vi "Generate Joint Trajectory (Int).vi"(4 "end joint velocities":dbl[](array[numeric]), 6 "start joint velocities":dbl[](array[numeric]), 7 "intermediate points":i32, 8 "error in (no error)":errorcluster, 10 "end joint positions":dbl[](array[numeric]), 11 "start joint positions":dbl[](array[numeric])) -> (0 "error out":errorcluster, 1 "joint acceleration trajectory":dbl[][](array[numeric]), 2 "joint velocity trajectory":dbl[][](array[numeric]), 3 "joint position trajectory":dbl[][](array[numeric]))   [LabVIEW 2017, in "NI_Kinematics.lvlib"]
doc: "Generates joint angles, velocities, and accelerations along a smooth trajectory between two points in joint space. Wire data to the <B>intermediate points</B> input to determine the polymorphic instance to use or manually select the instance.\n\n<B>.m file:</B> jtraj"
uses:
  <vilib>/robotics/Kinematics/NI_Kinematics.lvlib
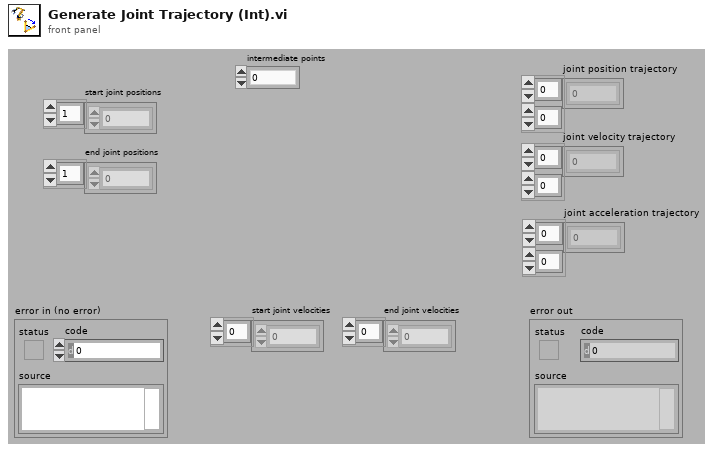
[diagram p1: front panel]
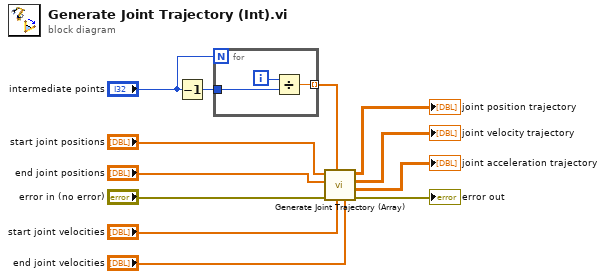
[diagram p0: block diagram]
diagram:
  n1 = Decrement(x="intermediate points") -> (x-1=w7:i32)
  n2 = for {
    N: "intermediate points" -> [_]
    tunnel: w7 -> [w15]
    tunnel: [w13] -> w5 mode=indexing
    i -> [w14]
    n3 = Divide(x=w14, y=w15) -> (x/y=w13:dbl)
  }
  n4 = call <vilib>:"Generate Joint Trajectory (Array).vi"("end joint velocities"="end joint velocities", "start joint velocities"="start joint velocities", "intermediate points"=w5, "error in (no error)"="error in (no error)", "end joint positions"="end joint positions", "start joint positions"="start joint positions") -> ("error out"=→"error out":errorcluster, "joint acceleration trajectory"=→"joint acceleration trajectory":dbl[][], "joint velocity trajectory"=→"joint velocity trajectory":dbl[][], "joint position trajectory"=→"joint position trajectory":dbl[][])  [unwired: 2 in]
